vi "Create Instance Impl.vi"(8 "error in (no error)":errorcluster, 10 "Configuration":T1, 11 "Thorlabs Power Meter in":refnum<class "Thorlabs Power Meter.lvclass">) -> (0 "error out":errorcluster, 3 "Thorlabs Power Meter out":refnum<class "Thorlabs Power Meter.lvclass">)   [LabVIEW 2023, in "Thorlabs Power Meter.lvlib" / "Thorlabs Power Meter.lvclass"]
uses:
  Thorlabs Power Meter.lvclass
  Thorlabs Power Meter.lvclass/Thorlabs Power Meter.ctl
  Thorlabs Power Meter.lvlib
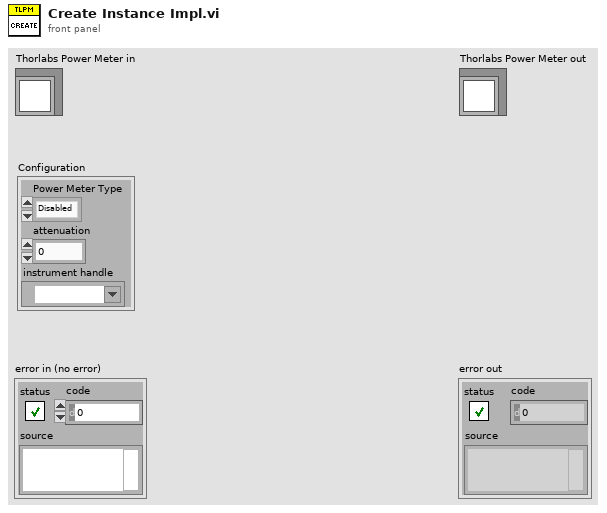
[diagram p1: front panel]
types:
  T1 = cluster{"Power Meter Type":enum16{"Disabled", "Thorlabs", "Newport", "Coherent"}, "attenuation":dbl, "instrument handle":refnum<visa-resource-name>}
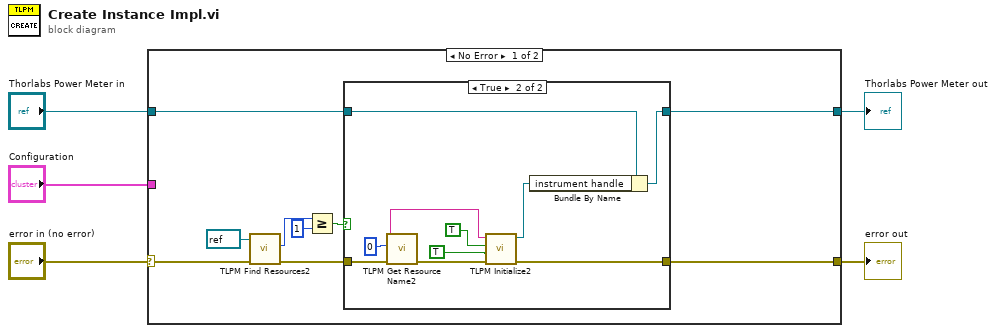
[diagram p0: block diagram]
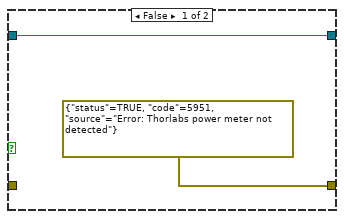
[diagram p2: hidden frame]
diagram:
  n1 = case shown="No Error" "error in (no error)" {
    selector: "error in (no error)" -> [w6 w27]
    tunnel: "Thorlabs Power Meter in" -> [w9 w28]
    tunnel: [w8 w28] -> w4
    tunnel: [w7 w27] -> w2
    tunnel: "Configuration" -> [_ _]
    frame No Error {
      n2 = call "TLPM Find Resources2.vi"("error in (no error)"=w6, "instrument handle"=refnum<visa-resource-name> refnum) -> ("error out"=w13:errorcluster, "Resource Count"=w14:u32)  [unwired: 7 in, 1 out]
      n3 = Greater Or Equal?(x=w14, y=u32 1) -> (x >= y?=w12:bool)
      n4 = case shown="True" w12 {
        tunnel: w13 -> [_ w26]
        tunnel: [errorcluster {"status"=TRUE, "code"=5951, "source"="Error: Thorlabs power meter not detected"} ("error constant") w23] -> w7
        tunnel: [w15 w18] -> w8
        tunnel: w9 -> [w15 w19]
        frame False {
        }
        frame True {
          n5 = call "TLPM Get Resource Name2.vi"("error in (no error)"=w26, "Index (0)"=u32 0 ("Device Index")) -> ("error out"=w24:errorcluster, "Resource Name"=w20:string)  [unwired: 7 in, 1 out]
          n6 = call "TLPM Initialize2.vi"("error in (no error)"=w24, "Reset Device (Reset Device)"=TRUE ("ID Query (Do Query)"), "ID Query (Do Query)"=TRUE, "resource name"=w20) -> ("error out"=w23:errorcluster, "instrument handle out"=w17:refnum<visa-resource-name>)  [unwired: 6 in]
          n7 = Bundle By Name(cluster=w19, "instrument handle"=w17) -> (w18:refnum<class "Thorlabs Power Meter.lvclass">)
        }
      }
    }
    frame Error {
    }
  }
  "error out" <- w2
  "Thorlabs Power Meter out" <- w4
